vi "Read Autostop Nested Actor Count.vi"(11 "Actor in":refnum<class "Actor.lvclass">) -> (2 "Count":i32)   [LabVIEW 2017, in "Actor Framework.lvlib" / "Actor.lvclass"]
doc: "This VI returns the number of auto-stop nested actors that were launched by this actor that have not yet sent back their Last Ack messages. You may use this VI to detect when all of this actor's nested actors have finished by seeing if this count has reached zero. Note that any nested actors launched with <b>Auto-stop?</b> set to false will not be included in this count; actors are responsible for counting those actors themselves."
uses:
  <vilib>/ActorFramework/Actor/Actor.lvclass
  <vilib>/ActorFramework/Actor/Actor.lvclass/Actor.ctl
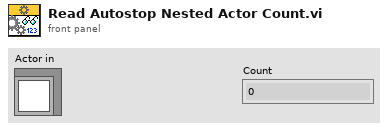
[diagram p1: front panel]
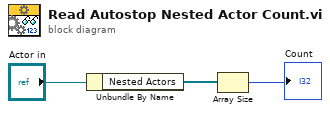
[diagram p0: block diagram]
diagram:
  n1 = Unbundle By Name("Actor in") -> ("Nested Actors"=w2:refnum<class "Message Enqueuer.lvclass">[])
  n2 = Array Size(array=w2) -> (size(s)=→"Count":i32)
